vi "Ports.vi"(0 "Test":string, 1 "Reserved array Input":string[](array[string])) -> (2 "Result Input":string[](array[string]), 3 "Ports counter":i32, 4 "Sizes":i32[](array[numeric]))   [LabVIEW 2012]
panel:
  out "before substring":string
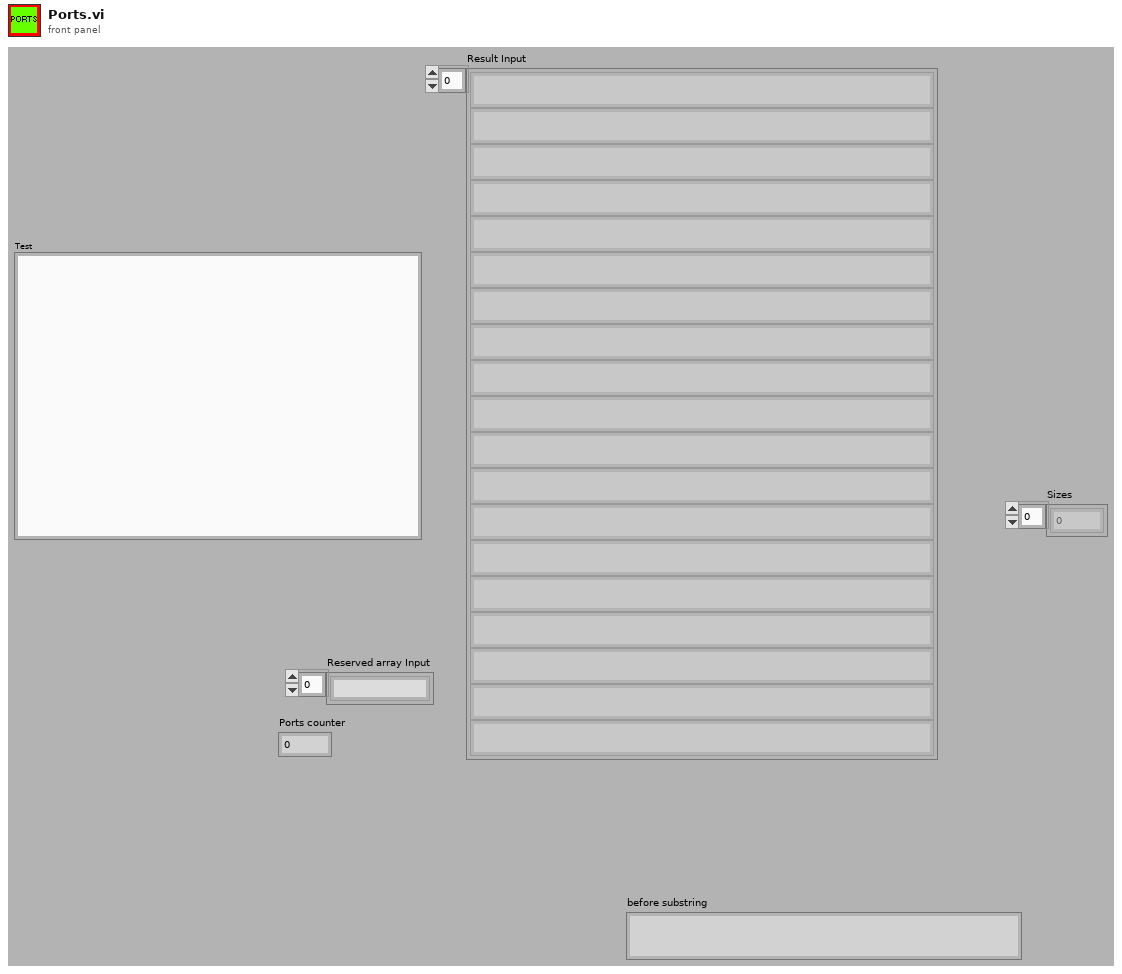
[diagram p1: front panel]
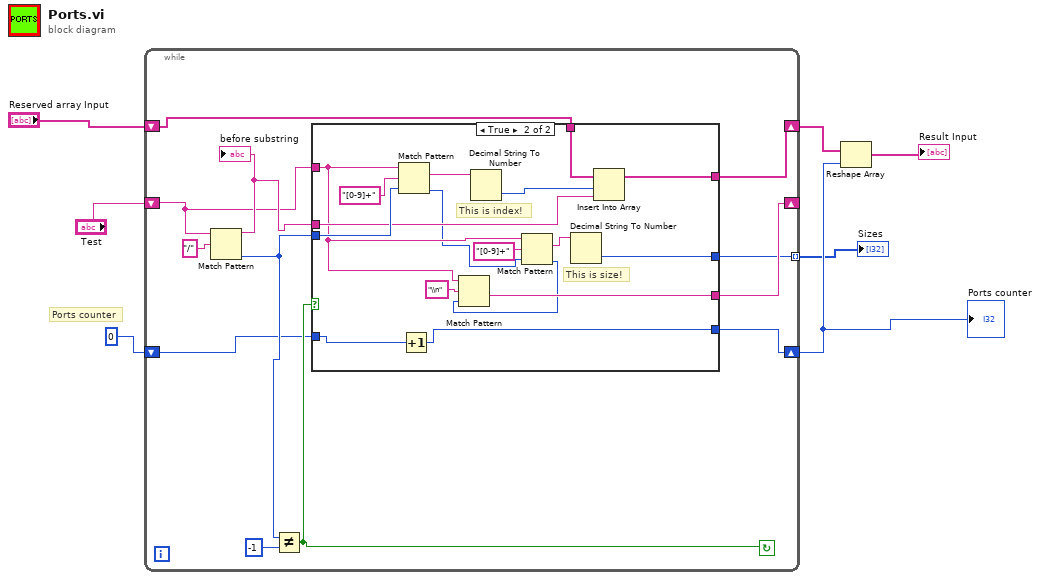
[diagram p0: block diagram]
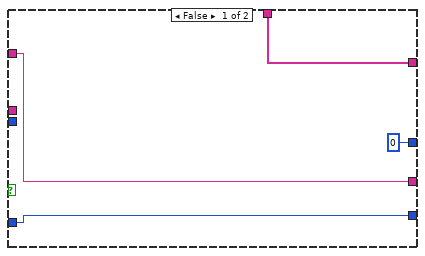
[diagram p2: hidden frame]
diagram:
  # "Ports counter"
  n1 = while {
    shift-right: [w14] -> w4
    shift-left: "Reserved array Input" -> [w16]
    shift-right: [w11] -> w2
    shift-left: 0 ("offset past match") -> [w12]
    shift-right: [w10] -> _
    shift-left: "Test" -> [w9]
    tunnel: [w8] -> w1 mode=indexing
    stop <- w13 continue-if-true
    n2 = Match Pattern(string=w9, regular expression="/" ("search string")) -> (before substring=w15:string, offset past match=w17:i32)  [unwired: 1 in, 2 out]
    "before substring" <- w15
    n3 = Not Equal?(x=w17, y=-1) -> (x != y?=w13:bool)
    n4 = case shown="True" w13 {
      tunnel: w9 -> [w21 w29]
      tunnel: w17 -> [_ w40]
      tunnel: w16 -> [w23 w37]
      tunnel: w15 -> [_ w35]
      tunnel: [w23 w34] -> w14
      tunnel: w12 -> [w22 w32]
      tunnel: [w22 w31] -> w11
      tunnel: [w21 w30] -> w10
      tunnel: [0 w24] -> w8
      frame False {
      }
      frame True {
        # "This is size!"
        # "This is index!"
        n5 = Match Pattern(string=w29, regular expression="[0-9]+", offset (0)=w40) -> (match substring=w38:string, offset past match=w27:i32)  [unwired: 2 out]
        n6 = Increment(x=w32) -> (x+1=w31:i32)
        n7 = Decimal String To Number(string=w38) -> (number=w36:i32)  [unwired: 2 in, 1 out]
        n8 = Match Pattern(string=w29, regular expression="[0-9]+", offset (0)=w27) -> (match substring=w26:string, offset past match=w25:i32)  [unwired: 2 out]
        n9 = Match Pattern(string=w29, regular expression="\\n" ("search string"), offset (0)=w25) -> (after substring=w30:string)  [unwired: 3 out]
        n10 = Decimal String To Number(string=w26) -> (number=w24:i32)  [unwired: 2 in, 1 out]
        n11 = Insert Into Array(array=w37, index=w36, new element=w35) -> (w34:string[])
      }
    }
  }
  "Ports counter" <- w2
  "Sizes" <- w1
  n12 = Reshape Array(w4, w2) -> (→"Result Input":string[])
